vi "OutputBallHandling.vi"   [LabVIEW 2019]
doc: "This VI runs feedback and feedforward control loops, manages safety interlocks, and sends commands to actuators specific to the intake, hopper, and magazine subsystem."
uses:
  <vilib>/Rock Robotics/WPI/Solenoid/WPI_SolenoidValue.ctl
  <vilib>/Rock Robotics/WPI/ThirdParty/Phoenix-LabVIEW/Motor Controller/Controls/CTRE_Phoenix_MotorControl_ControlMode.ctl
  3907ee5d-d888-435e-9563-35184685acb4.vi
  86fbdfb1-fed5-4583-8cdc-41b9d6d948da.vi
  f5708eb5-0e7b-4c1b-96ce-dc5ca0a5594e.vi
  refnums.vi
  GRNF_CTREMotor.vi
  GRNF_GenericSolenoid.vi
  outputs.vi
  TAI_Motor.vi
  dsdata.vi
  TAI_Solenoid.vi
  <vilib>/Rock Robotics/WPI/Solenoid/WPI_SolenoidSetEnum.vi
types:
  T1 = typedef "WPI_SolenoidDevRef.ctl" = cluster{"DevStatus":errorcluster, "Pneumatics Control Module":u8, "Forward Solenoid Channel":T2, "Reverse Solenoid Channel":T2}
  T2 = typedef "WPI_SolenoidChannel.ctl" = enum8{"Solenoid 0", "Solenoid 1", "Solenoid 2", "Solenoid 3", "Solenoid 4", "Solenoid 5", "Solenoid 6", "Solenoid 7", "Invalid"}
  T3 = typedef "WPI_MotorControlDeviceRef.ctl" = cluster{"DeviceStatus":errorcluster, "Type":T4, "PWM":cluster{"PWM Channel":T5, "DeadBand":T6}, "CAN":cluster{"Device Number":u8, "SetOutput VI Ref":variant, "GetOutput VI Ref":variant, "Enable VI Ref":variant, "Disable VI Ref":variant, "Data":variant}, "Invert":bool, "DIO PWM":cluster{"PWM \"Enable\" Channel":T5, "DIOChannel":T7, "PWM Rate":dbl}}
  T4 = typedef "WPI_MotorControlType.ctl" = enum16{"PWM", "CAN", "DIO PWM"}
  T5 = typedef "FPGA_DIOPWMChannel.ctl" = enum8{"PWM 0", "PWM 1", "PWM 2", "PWM 3", "PWM 4", "PWM 5", "PWM 6", "PWM 7", "PWM 8", "PWM 9", "PWM MXP 0", "PWM MXP 1", "PWM MXP 2", "PWM MXP 3", "PWM MXP 4", "PWM MXP 5", "PWM MXP 6", "PWM MXP 7", "PWM MXP 8", "PWM MXP 9", "Invalid"}
  T6 = typedef "WPI_PWMDeadband.ctl" = cluster{"Name":string, "maxPositivePwm":i32, "minPositivePwm":i32, "centerPwm":i32, "maxNegativePwm":i32, "minNegativePwm":i32, "angularRange":u16}
  T7 = typedef "FPGA_DIOChannel.ctl" = enum8{"DIO 0", "DIO 1", "DIO 2", "DIO 3", "DIO 4", "DIO 5", "DIO 6", "DIO 7", "DIO 8", "DIO 9", "DIO MXP 0", "DIO MXP 1", "DIO MXP 2", "DIO MXP 3", "DIO MXP 4", "DIO MXP 5", "DIO MXP 6", "DIO MXP 7", "DIO MXP 8", "DIO MXP 9", "DIO MXP 10", "DIO MXP 11", "DIO MXP 12", "DIO MXP 13", "DIO MXP 14", "DIO MXP 15", "SPI Port CS1", "SPI Port CS2", "SPI Port CS3", "SPI Port MISO", "SPI Port MOSI", "Invalid"}
  T8 = typedef "WPI_SolenoidValue.ctl" = enum16{"Off", "On", "Forward", "Reverse"}
  T9 = typedef "CTRE_Phoenix_MotorControl_ControlMode.ctl" = u16
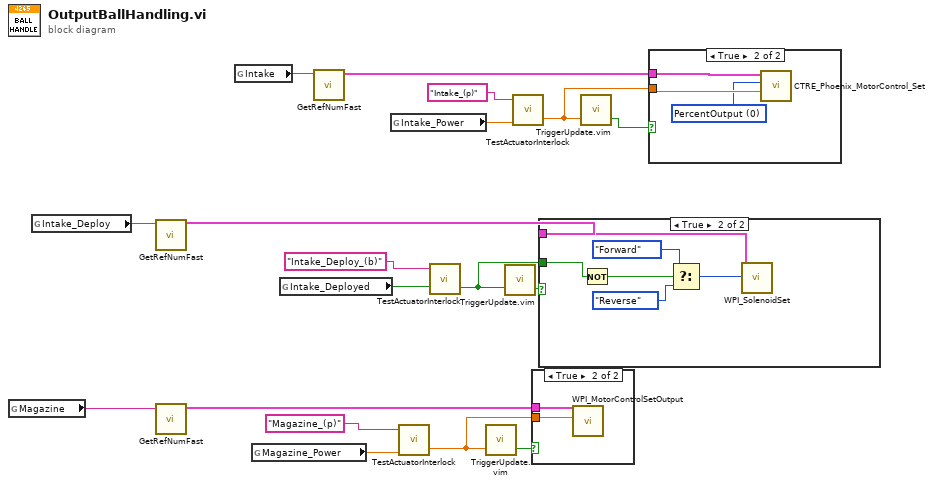
[diagram p0: block diagram]
diagram:
  n1 = global read "refnums.vi" "Magazine"() -> (w15:string)
  n2 = global read "refnums.vi" "Intake_Deploy"() -> (w17:string)
  n3 = call-poly "GetRefNumFast.vi"("RefNum Name"=w17) -> ("Device Reference"=w1:T1)  [unwired: 5 in, 1 out]
  n4 = call-poly "GetRefNumFast.vi"("RefNum Name"=w15) -> ("Device Reference"=w16:T3)  [unwired: 5 in, 1 out]
  n5 = global read "refnums.vi" "Intake"() -> (w18:string)
  n6 = global read "outputs.vi" "Magazine_Power"() -> (w13:dbl)
  n7 = global read "outputs.vi" "Intake_Deployed"() -> (w4:bool)
  n8 = call-poly "GetRefNumFast.vi"("RefNum Name"=w18) -> ("Device Reference"=w8:T3)  [unwired: 5 in, 1 out]
  n9 = global read "outputs.vi" "Intake_Power"() -> (w9:dbl)
  n10 = call-poly "TestActuatorInterlock.vi"("Normal Output"=w13, "Actuator Name"="Magazine_(p)" ("Actuator_Name")) -> ("Interlock Output"=w11:dbl)  [unwired: 1 in, 1 out]
  n11 = call-poly "TestActuatorInterlock.vi"("Normal Output"=w4, "Actuator Name"="Intake_Deploy_(b)" ("Actuator_Name")) -> ("Interlock Output"=w2:bool)  [unwired: 1 in, 1 out]
  n12 = call "TriggerUpdate.vim"("Trigger"=w11) -> ("Update"=w12:bool)  [unwired: 2 in]
  n13 = call "TriggerUpdate.vim"("Trigger"=w2) -> ("Update"=w3:bool)  [unwired: 2 in]
  n14 = call-poly "TestActuatorInterlock.vi"("Normal Output"=w9, "Actuator Name"="Intake_(p)" ("Actuator_Name")) -> ("Interlock Output"=w6:dbl)  [unwired: 1 in, 1 out]
  n15 = case shown="True" w12 {
    tunnel: w16 -> [_ w20]
    tunnel: w11 -> [_ w19]
    frame False {
    }
    frame True {
      n16 = call <vilib>:"WPI_MotorControlSetOutput.vi"("Output"=w19, "MotorControlDevRef"=w20) -> ()  [unwired: 7 in, 3 out]
    }
  }
  n17 = case shown="True" w3 {
    tunnel: w2 -> [_ w25]
    tunnel: w1 -> [_ w26]
    frame False {
    }
    frame True {
      n18 = Not(x=w25) -> (.not. x?=w21:bool)
      n19 = Select(t=WPI_SolenoidValue."Forward" ("Value"), s=w21, f=WPI_SolenoidValue."Reverse" ("Value")) -> (s? t:f=w22:T8)
      n20 = call-poly <vilib>:"WPI_SolenoidSet.vi"("Value"=w22, "SolenoidDevRef"=w26) -> ()  [unwired: 8 in, 2 out]
    }
  }
  n21 = call "TriggerUpdate.vim"("Trigger"=w6) -> ("Update"=w7:bool)  [unwired: 2 in]
  n22 = case shown="True" w7 {
    tunnel: w8 -> [_ w29]
    tunnel: w6 -> [_ w28]
    frame False {
    }
    frame True {
      w27 = T9 0 items=["PercentOutput"=0, "Position"=1, "Velocity"=2, "Current"=3, "Follower"=5, "MotionProfile"=6, "MotionMagic"=7, "MotionProfileArc"=10, "Disabled"=15] ("Control Mode")
      n23 = call <vilib>:"CTRE_Phoenix_MotorControl_Set.vi"("Output"=w28, "Control Mode"=w27, "PhoenixMotorControlDevRef"=w29) -> ()  [unwired: 7 in, 2 out]
    }
  }
